vi "teste-motor-2.vi"() -> ()   [LabVIEW 2014]
uses:
  C:/user-Lab/AndreTec/GITs/andretec/Thorlabs-Vector-Move/kinesisTec/Kinesis/Thorlabs.MotionControl.Controls.dll
  kinesisTec/Kinesis/Thorlabs.MotionControl.Controls.dll
  C:/user-Lab/AndreTec/GITs/andretec/Thorlabs-Vector-Move/kinesisTec/Kinesis/Thorlabs.MotionControl.TCube.DCServoCLI.dll
  kinesisTec/Kinesis/Thorlabs.MotionControl.TCube.DCServoCLI.dll
  C:/user-Lab/AndreTec/GITs/andretec/Thorlabs-Vector-Move/kinesisTec/Kinesis/Thorlabs.MotionControl.GenericMotorCLI.dll
  kinesisTec/Kinesis/Thorlabs.MotionControl.GenericMotorCLI.dll
panel:
  in  "position":dbl
  out "Acc 2":dbl
  out "MinVelocity":dbl
  out "MaxVelocity 2":dbl
  in  "stop 2":bool
  in  "MaxVelocity":dbl=2.2
  in  "Acceleration":dbl=1.5
  out "x/y":dbl=4.015304337686567
  in  "stop":bool
  in  "TCubeDCServoControl":refnum<k24>(container)
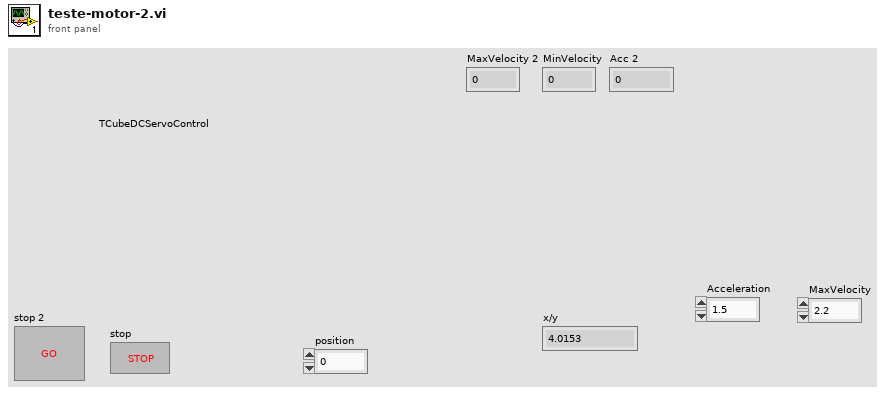
[diagram p1: front panel]
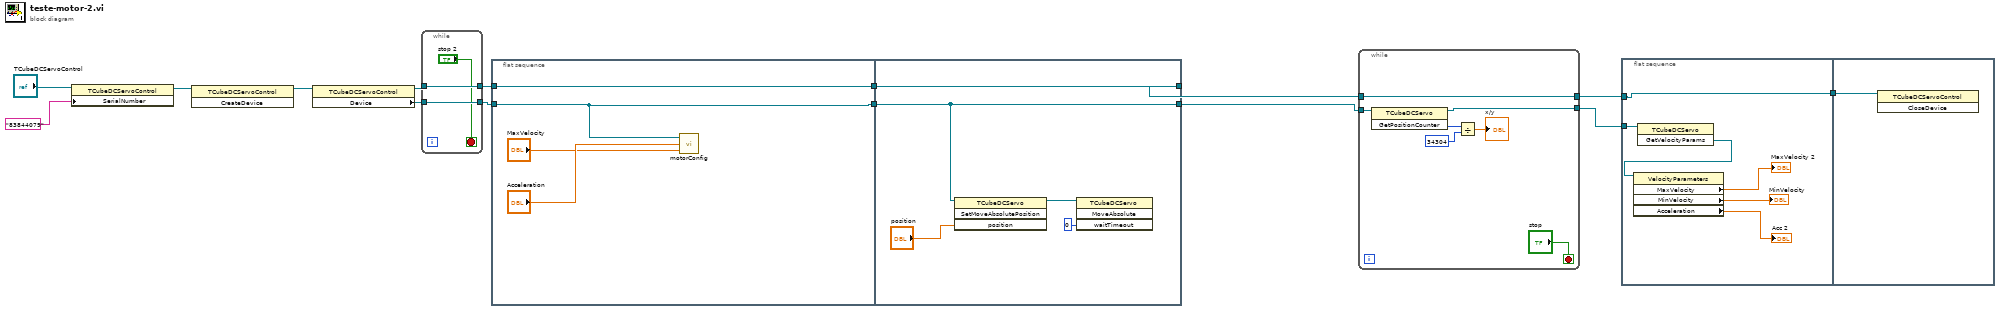
[diagram p0: block diagram]
diagram:
  n1 = property class="TCubeDCServoControl"(reference="TCubeDCServoControl", "SerialNumber"="83844079") -> (reference out=w13:refnum<k24>)  [unwired: 1 in, 1 out]
  n2 = invoke class="TCubeDCServoControl" method="CreateDevice"(reference=w13) -> (reference out=w12:refnum<k24>)  [unwired: 2 in, 2 out]
  n3 = property class="TCubeDCServoControl"(reference=w12) -> (reference out=w11:refnum<k24>, "Device"=w10:refnum<k24>)  [unwired: 1 in, 1 out]
  n4 = while {
    tunnel: [w18] -> w5
    tunnel: w11 -> [w18]
    tunnel: w10 -> [w17]
    tunnel: [w17] -> w6
    stop <- "stop 2" stop-if-true
  }
  n5 = flat-sequence {
    tunnel: w6 -> [w19]
    tunnel: w5 -> [w20]
    tunnel: [w20] -> w2
    tunnel: [w19] -> w1
    tunnel: [w23] -> w3
    tunnel: [w27] -> w4
    tunnel: w2 -> [w27]
    tunnel: w1 -> [w23]
    frame #0 {
      n6 = call "motorConfig.vi"("Velocity"="MaxVelocity", "Acceleration"="Acceleration", "Device in"=w19) -> ()  [unwired: 2 in, 1 out]
    }
    frame #1 {
      n7 = invoke class="TCubeDCServo" method="SetMoveAbsolutePosition"(reference=w23, "position"="position") -> (reference out=w24:refnum<k24>)  [unwired: 2 in, 3 out]
      n8 = invoke class="TCubeDCServo" method="MoveAbsolute"(reference=w24, "waitTimeout"=0) -> ()  [unwired: 2 in, 4 out]
    }
  }
  n9 = while {
    tunnel: w4 -> [w33]
    tunnel: [w33] -> w8
    tunnel: w3 -> [w32]
    tunnel: [w28] -> w9
    stop <- "stop" stop-if-true
    n10 = invoke class="TCubeDCServo" method="GetPositionCounter"(reference=w32) -> (reference out=w28:refnum<k24>, "GetPositionCounter"=w31:i32)  [unwired: 2 in, 1 out]
    n11 = Divide(x=w31, y=34304) -> (x/y=→"x/y":dbl)
  }
  n12 = flat-sequence {
    tunnel: w9 -> [w36]
    tunnel: [w35] -> _
    tunnel: w8 -> [w35]
    tunnel: [w35] -> w7
    tunnel: w7 -> [w41]
    frame #0 {
      n13 = invoke class="TCubeDCServo" method="GetVelocityParams"(reference=w36) -> ("GetVelocityParams"=w40:refnum<k24>)  [unwired: 2 in, 2 out]
      n14 = property class="VelocityParameters"(reference=w40) -> ("MaxVelocity"=→"MaxVelocity 2":dbl, "MinVelocity"=→"MinVelocity":dbl, "Acceleration"=→"Acc 2":dbl)  [unwired: 1 in, 2 out]
    }
    frame #1 {
      n15 = invoke class="TCubeDCServoControl" method="CloseDevice"(reference=w41) -> ()  [unwired: 2 in, 3 out]
    }
  }
